vi "Set frequency.vi"(8 "error in (no error)":errorcluster, 10 "frequency":dbl=5180000000.0 format="%#_6p", 11 "niDTS WLAN Dut in":refnum<class "niDTS WLAN Dut.lvclass">) -> (0 "error out":errorcluster, 3 "niDTS WLAN Dut out":refnum<class "niDTS WLAN Dut.lvclass">)   [LabVIEW 2015, in "niDTS WLAN.lvlib" / "niDTS WLAN Dut.lvclass"]
uses:
  niDTS WLAN Dut.lvclass
  niDTS WLAN Dut.lvclass/niDTS WLAN Dut.ctl
  niDTS WLAN.lvlib
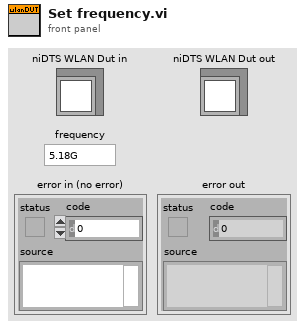
[diagram p1: front panel]
types:
  T1 = typedef "niDTS WLAN.lvlib/niDTS WLAN INC CH BW.ctl" = enum16{"20 MHz", "40 MHz", "80 MHz", "160 MHz"}
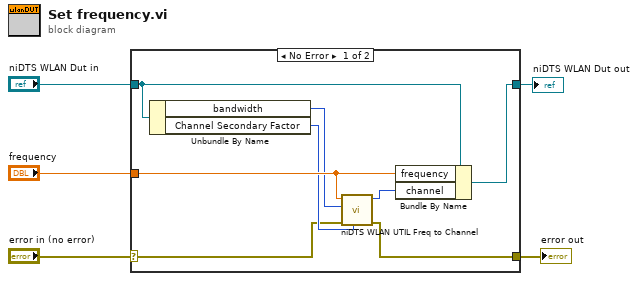
[diagram p0: block diagram]
diagram:
  n1 = case shown="No Error" "error in (no error)" {
    selector: "error in (no error)" -> [w8 w14]
    tunnel: [w7 w14] -> w4
    tunnel: [w13 w15] -> w2
    tunnel: "niDTS WLAN Dut in" -> [w12 w15]
    tunnel: "frequency" -> [w11 _]
    frame No Error {
      n2 = Unbundle By Name(w12) -> ("bandwidth"=w10:T1, "Channel Secondary Factor"=w9:i8)
      n3 = call "niDTS WLAN UTIL Freq to Channel.vi"("secondary factor"=w9, "error in"=w8, "CH BW"=w10, "Center Frequency"=w11) -> ("error out"=w7:errorcluster, "Channel"=w6:u32)  [unwired: 6 in]
      n4 = Bundle By Name(cluster=w12, "frequency"=w11, "channel"=w6) -> (w13:refnum<class "niDTS WLAN Dut.lvclass">)
    }
    frame Error {
    }
  }
  "error out" <- w4
  "niDTS WLAN Dut out" <- w2
